vi "ParameterSet2DesiredParameters.vi"(7 "ParameterSet":string) -> (4 "DesiredParameters":T1)   [LabVIEW 2013]
uses:
  TypeDef/Command Cluster.ctl
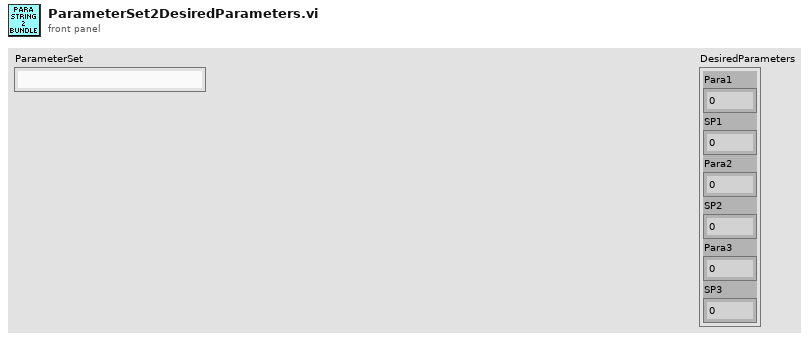
[diagram p1: front panel]
types:
  T1 = typedef "Command Cluster.ctl" = cluster{"Para1":i32, "SP1":dbl, "Para2":i32, "SP2":dbl, "Para3":i32, "SP3":dbl}
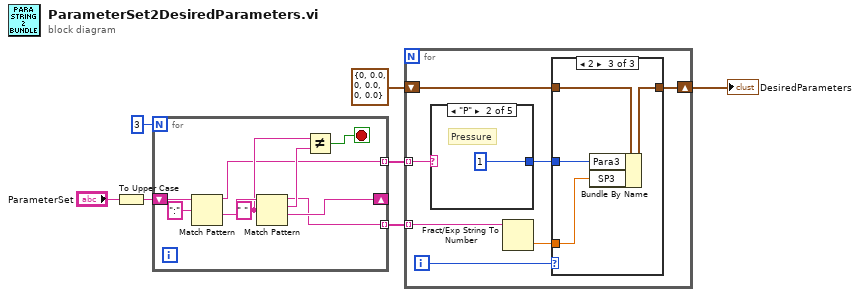
[diagram p0: block diagram]
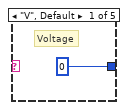
[diagram p2: hidden frame]
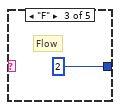
[diagram p3: hidden frame]
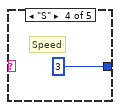
[diagram p4: hidden frame]
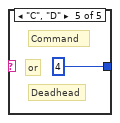
[diagram p5: hidden frame]
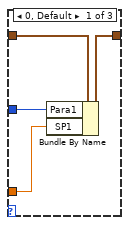
[diagram p6: hidden frame]
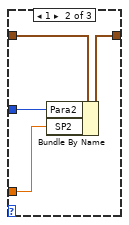
[diagram p7: hidden frame]
diagram:
  n1 = To Upper Case(1:"ParameterSet") -> (0:w3:string)
  n2 = for {
    N: 3 -> [_]
    shift-right: [w9] -> _
    shift-left: w3 -> [w16]
    tunnel: [w8] -> w2 mode=indexing
    tunnel: [w10] -> w4 mode=indexing
    stop <- w11 stop-if-true
    w13 = " " ("regular expression")
    n3 = Match Pattern(string=w16, regular expression=":") -> (before substring=w10:string, after substring=w14:string)  [unwired: 1 in, 2 out]
    n4 = Match Pattern(string=w14, regular expression=w13) -> (before substring=w8:string, match substring=w12:string, after substring=w9:string)  [unwired: 1 in, 1 out]
    n5 = Not Equal?(x=w13, y=w12) -> (x != y?=w11:bool)
  }
  n6 = for {
    tunnel: w2 -> [w22] mode=indexing
    tunnel: w4 -> [w20] mode=indexing
    shift-right: [w18] -> w6
    shift-left: T1 {"Para1"=0, "SP1"=0.0, "Para2"=0, "SP2"=0.0, "Para3"=0, "SP3"=0.0} ("CMDCluster In") -> [w19]
    i -> [w23]
    n7 = case shown="\"P\"" w20 {
      tunnel: [0 ("Para1") 1 ("Para1") 2 ("Para1") 3 ("Para1") 4 ("Para1")] -> w17
      frame "V", Default {
        # "Voltage"
      }
      frame "P" {
        # "Pressure"
      }
      frame "F" {
        # "Flow"
      }
      frame "S" {
        # "Speed"
      }
      frame "C", "D" {
        # "or"
        # "Deadhead"
        # "Command"
      }
    }
    n8 = Fract/Exp String To Number(string=w22) -> (number=w21:dbl)  [unwired: 3 in, 1 out]
    n9 = case shown="2" w23 {
      tunnel: w21 -> [w29 w33 w37]
      tunnel: w19 -> [w32 w36 w40]
      tunnel: [w31 w35 w39] -> w18
      tunnel: w17 -> [w30 w34 w38]
      frame 0, Default {
        n10 = Bundle By Name(cluster=w32, "Para1"=w30, "SP1"=w29) -> (w31:T1)
      }
      frame 1 {
        n11 = Bundle By Name(cluster=w36, "Para2"=w34, "SP2"=w33) -> (w35:T1)
      }
      frame 2 {
        n12 = Bundle By Name(cluster=w40, "Para3"=w38, "SP3"=w37) -> (w39:T1)
      }
    }
  }
  "DesiredParameters" <- w6
